vi "Localization.vi"(11 "未本地化":string) -> (3 "本地化":string)   [LabVIEW 2013, in "Air Cooler Application.lvlib" / "Air Cooler Application.lvclass"]
doc: "本VI用于本地化支持，支持其他语言的用户界面。对于给定的输入字符串，本VI按当前语言返回该字符串的翻译。开发人员可以通过LabVIEW的“导出/导入字符串”功能生成一个可翻译的文件。按照规范，带“DNL_”标签的控件不会被翻译（在英语中，DNL表示不要本地化）。本VI的第一个数组就是一个DNL_控件。该数组中包含程序所用的固定字符串。第二个数组包含翻译后的字符串。用这种方法处理用户可见的所有文本对于程序员来说优势很麻烦，但这样做可以限制本地化人员需要检查的VI数量。\n\n即便不需要翻译为其他语言，这种字符串查询的设计为用户可见的所有文本提供了一个集中存放的位置，便于在程序中多处复用，也便于技术文档撰写人员检查拼写错误，并将在开发周期的最后阶段修改拼写错误从而影响其他代码的风险最小化。"
uses:
  Air Cooler Application.lvclass
panel:
  in  "DNL_Unlocalized Array":string[](array[string])=["Stop All"]
  in  "已本地化数组":string[](array[string])=["停止全部"]
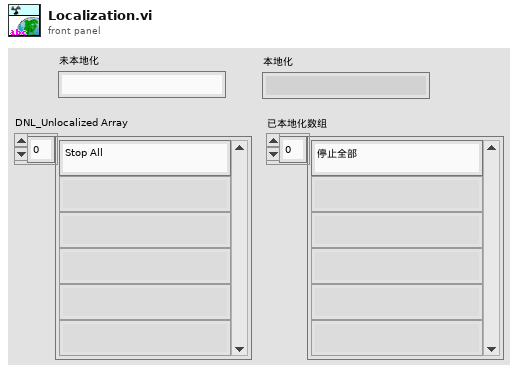
[diagram p1: front panel]
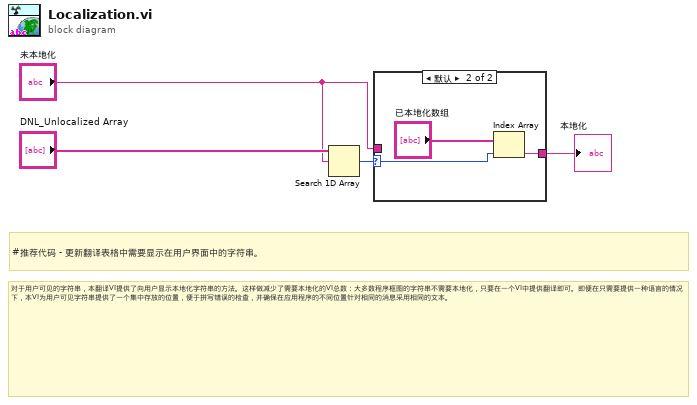
[diagram p0: block diagram]
diagram:
  # "#推荐代码 - 更新翻译表格中需要显示在用户界面中的字符串。"
  # "对于用户可见的字符串，本翻译VI提供了向用户显示本地化字符串的方法。这样做减少了需要本地化的VI总数：大多数程序框图的字符串不需要本地化，只要在一个VI中提供翻译即可。即便在只需要提供一种语言的情况下，本VI为用户可见字符串提供了一个集中存放的位置，便于拼写错误的检查，并确保在应用程序的不同位置针对相同的消息采用相同的文本。"
  n1 = Search 1D Array(1D array="DNL_Unlocalized Array", element="未本地化") -> (index of element=w2:i32)  [unwired: 1 in]
  n2 = case shown="默认" w2 {
    selector: w2 -> [_ w6]
    tunnel: [w5 w7] -> w3
    tunnel: "未本地化" -> [w5 _]
    frame ..-1 {
    }
    frame Default {
      n3 = Index Array(array="已本地化数组", index=w6) -> (element=w7:string)
    }
  }
  "本地化" <- w3
